vi "down string pot slow.vi"(10 "Joystick Axis":dbl) -> (1 "motor output":dbl)   [LabVIEW 2014]
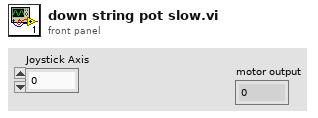
[diagram p1: front panel]
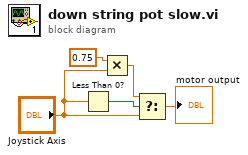
[diagram p0: block diagram]
diagram:
  n1 = Less Than 0?(x="Joystick Axis") -> (x < 0?=w5:bool)
  n2 = Multiply(x=0.75, y="Joystick Axis") -> (x*y=w3:dbl)
  n3 = Select(t=w3, s=w5, f="Joystick Axis") -> (s? t:f=→"motor output":dbl)
